vi "acquire_ShootDualTalonSrx.vi"(8 "error in":errorcluster, 11 "QuadTalonSRXDriveRef":T1={"LeftMasterDriveRef"={"DeviceStatus"={"status"=FALSE, "code"=0, "source"=""}, "Type"=enum."PWM", "PWM"={"PWM Channel"=enum."Invalid", "DeadBand"={"Name"="", "maxPositivePwm"=0, "minPositivePwm"=0, "centerPwm"=0, "maxNegativePwm"=0, "minNegativePwm"=0, "angularRange"=0}}, "CAN"={"Device Number"=0, "SetOutput VI Ref"=variant(refnum<vi> refnum), "GetOutput VI Ref"=variant(refnum<vi> refnum), "Enable VI Ref"=variant(refnum<vi> refnum), "Disable VI Ref"=variant(refnum<vi> refnum), "Data"=variant}, "Invert"=FALSE, "DIO PWM"={"PWM \"Enable\" Channel"=enum."Invalid", "DIOChannel"=enum."Invalid", "PWM Rate"=0.0}}, "RightMasterDriveRef"={"DeviceStatus"={"status"=FALSE, "code"=0, "source"=""}, "Type"=enum."PWM", "PWM"={"PWM Channel"=enum."Invalid", "DeadBand"={"Name"="", "maxPositivePwm"=0, "minPositivePwm"=0, "centerPwm"=0, "maxNegativePwm"=0, "minNegativePwm"=0, "angularRange"=0}}, "CAN"={"Device Number"=0, "SetOutput VI Ref"=variant(refnum<vi> refnum), "GetOutput VI Ref"=variant(refnum<vi> refnum), "Enable VI Ref"=variant(refnum<vi> refnum), "Disable VI Ref"=variant(refnum<vi> refnum), "Data"=variant}, "Invert"=FALSE, "DIO PWM"={"PWM \"Enable\" Channel"=enum."Invalid", "DIOChannel"=enum."Invalid", "PWM Rate"=0.0}}}) -> (0 "error out":errorcluster)   [LabVIEW 2019, in "ShootDualTalonSRX_Motor_Pair.lvlib"]
doc: "This VI is called for each TeleOp packet received from the DS where the robot is not disabled. It is often used to read from the joysticks and update I/O or to update setpoints for timed control loops. It should complete and return within 20 milliseconds or it may miss DS packets."
uses:
  ShootDualTalonSRX_Motor_Pair.lvlib
  <vilib>/Rock Robotics/WPI/ThirdParty/Phoenix-LabVIEW/Motor Controller/Get/CTRE_Phoenix_MotorController_GetSelectedSensorData.vi
  <vilib>/Rock Robotics/WPI/ThirdParty/Phoenix-LabVIEW/Motor Controller/Get/CTRE_Phoenix_MotorController_GetVoltage.vi
  globals_ShootDualTalonSRX.vi
  <vilib>/Rock Robotics/SystemInterfaces/DIO/FPGA_DIOPWMChannel.ctl
  <vilib>/Rock Robotics/WPI/PWM/WPI_PWMDeadband.ctl
  <vilib>/Rock Robotics/WPI/MotorControl/WPI_MotorControlType.ctl
  <vilib>/Rock Robotics/SystemInterfaces/DIO/FPGA_DIOChannel.ctl
  <vilib>/Rock Robotics/WPI/MotorControl/WPI_MotorControlDeviceRef.ctl
  ctrlRef_ShootDualTalon.ctl
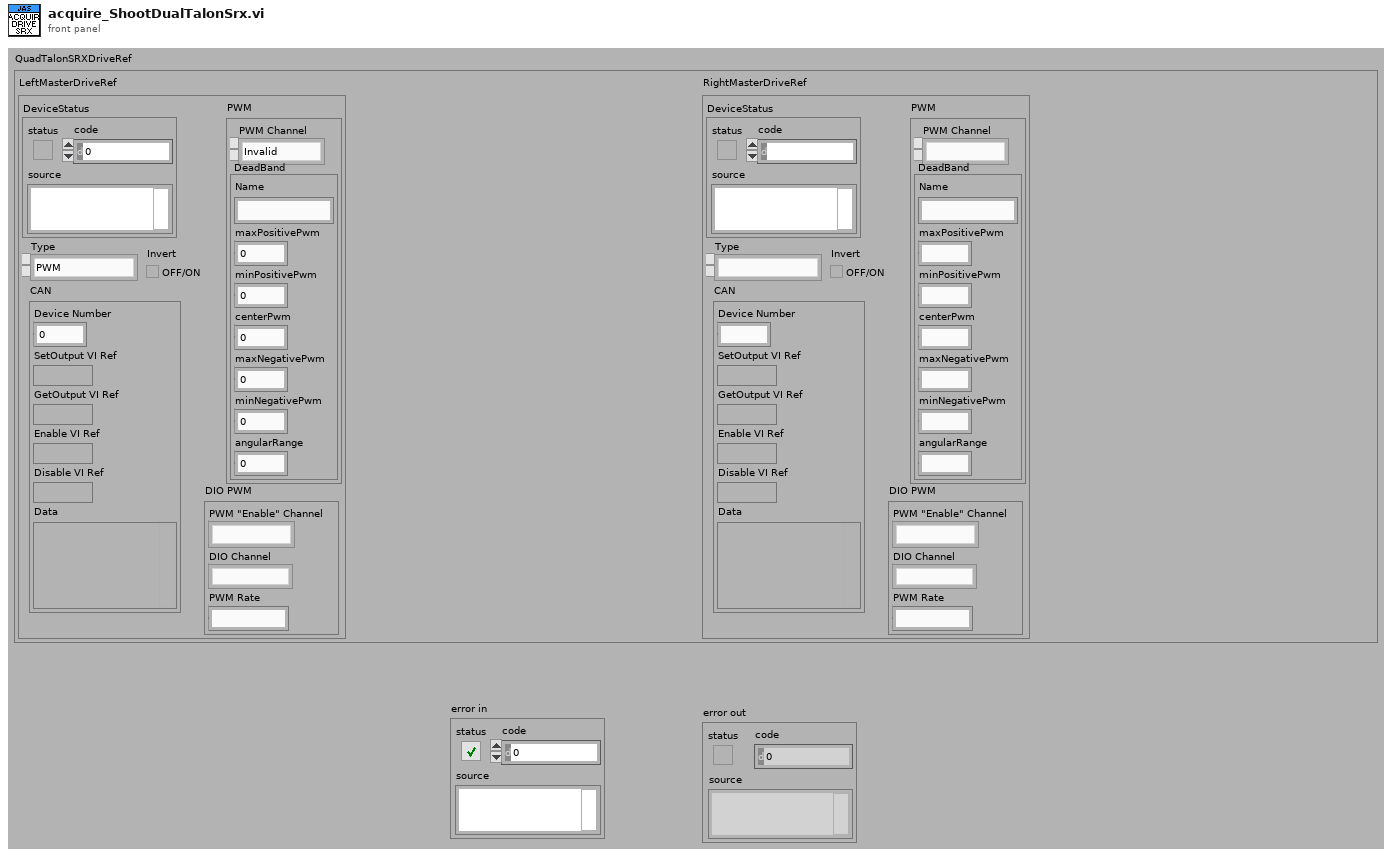
[diagram p1: front panel]
types:
  T1 = typedef "ShootDualTalonSRX_Motor_Pair.lvlib/ctrlRef_ShootDualTalon.ctl" = cluster{"LeftMasterDriveRef":T2, "RightMasterDriveRef":T2}
  T2 = typedef "WPI_MotorControlDeviceRef.ctl" = cluster{"DeviceStatus":errorcluster, "Type":T3, "PWM":cluster{"PWM Channel":T4, "DeadBand":T5}, "CAN":cluster{"Device Number":u8, "SetOutput VI Ref":variant, "GetOutput VI Ref":variant, "Enable VI Ref":variant, "Disable VI Ref":variant, "Data":variant}, "Invert":bool, "DIO PWM":cluster{"PWM \"Enable\" Channel":T4, "DIOChannel":T6, "PWM Rate":dbl}}
  T3 = typedef "WPI_MotorControlType.ctl" = enum16{"PWM", "CAN", "DIO PWM"}
  T4 = typedef "FPGA_DIOPWMChannel.ctl" = enum8{"PWM 0", "PWM 1", "PWM 2", "PWM 3", "PWM 4", "PWM 5", "PWM 6", "PWM 7", "PWM 8", "PWM 9", "PWM MXP 0", "PWM MXP 1", "PWM MXP 2", "PWM MXP 3", "PWM MXP 4", "PWM MXP 5", "PWM MXP 6", "PWM MXP 7", "PWM MXP 8", "PWM MXP 9", "Invalid"}
  T5 = typedef "WPI_PWMDeadband.ctl" = cluster{"Name":string, "maxPositivePwm":i32, "minPositivePwm":i32, "centerPwm":i32, "maxNegativePwm":i32, "minNegativePwm":i32, "angularRange":u16}
  T6 = typedef "FPGA_DIOChannel.ctl" = enum8{"DIO 0", "DIO 1", "DIO 2", "DIO 3", "DIO 4", "DIO 5", "DIO 6", "DIO 7", "DIO 8", "DIO 9", "DIO MXP 0", "DIO MXP 1", "DIO MXP 2", "DIO MXP 3", "DIO MXP 4", "DIO MXP 5", "DIO MXP 6", "DIO MXP 7", "DIO MXP 8", "DIO MXP 9", "DIO MXP 10", "DIO MXP 11", "DIO MXP 12", "DIO MXP 13", "DIO MXP 14", "DIO MXP 15", "SPI Port CS1", "SPI Port CS2", "SPI Port CS3", "SPI Port MISO", "SPI Port MOSI", "Invalid"}
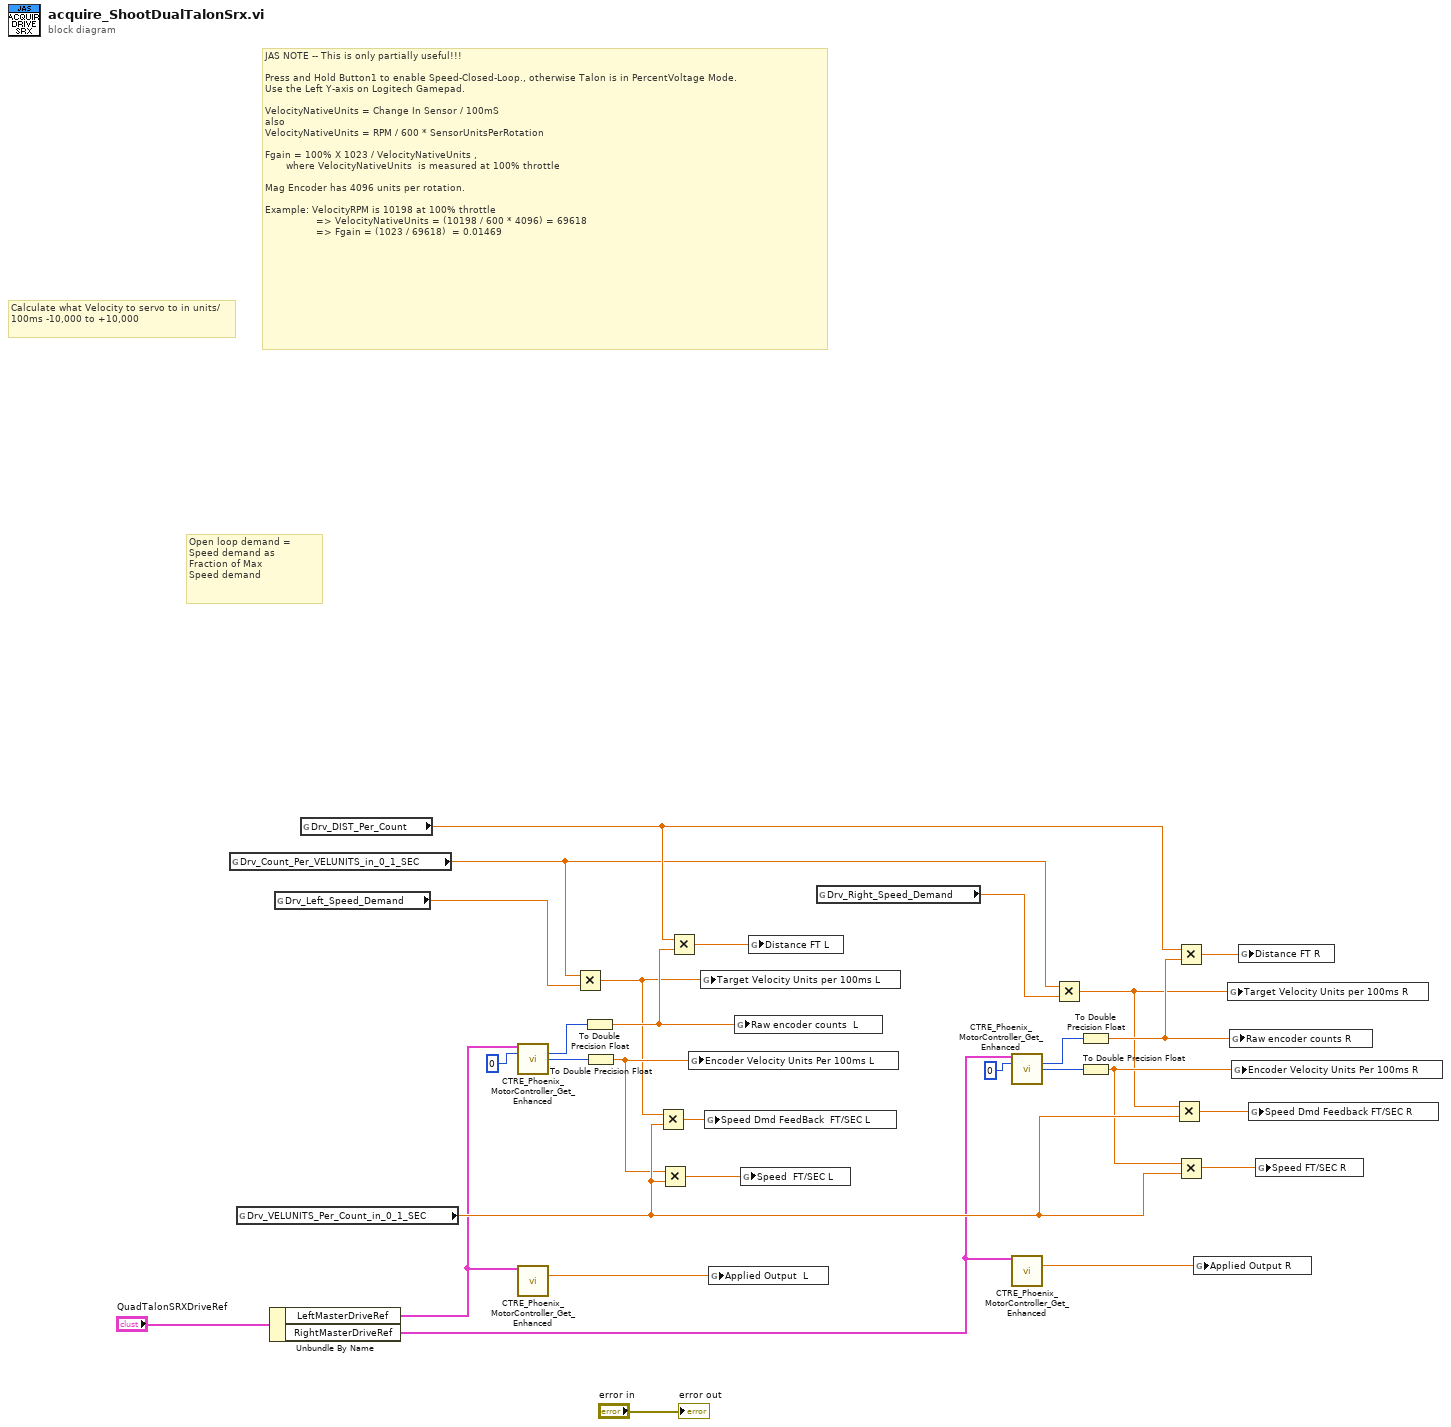
[diagram p0: block diagram]
diagram:
  # "Open loop demand = \nSpeed demand as\nFraction of Max\nSpeed demand"
  # "JAS NOTE -- This is only partially useful!!!\n\nPress and Hold Button1 to enable Speed-Closed-Loop., otherwise Talon is in PercentVoltage Mode.  \nUse the Left Y-axis on Logitech Gamepad.\n\nVelocityNativeUnits = Change In Sensor / 100mS\nalso\nVelocityNativeUnits = RPM / 600 * SensorUnitsPerRotation\n\nFgain = 100% X 1023 / VelocityNativeUnits , \n       where VelocityNativeUnits  is measured at 100% throttle\n\nMag Encoder has 4096 units per rotation.\n\nExample: VelocityRPM is 10198 at 100% throttle\n                 => VelocityNativeUnits = (10198 / 600 * 4096) = 69618\n                 => Fgain = (1023 / 69618)  = 0.01469"
  # "Calculate what Velocity to servo to in units/100ms -10,000 to +10,000"
  n1 = global read "globals_ShootDualTalonSRX.vi" "Drv_Count_Per_VELUNITS_in_0_1_SEC"() -> (w17:dbl)
  n2 = global read "globals_ShootDualTalonSRX.vi" "Drv_VELUNITS_Per_Count_in_0_1_SEC"() -> (w21:dbl)
  n3 = Unbundle By Name("QuadTalonSRXDriveRef") -> ("LeftMasterDriveRef"=w20:T2, "RightMasterDriveRef"=w19:T2)
  n4 = global read "globals_ShootDualTalonSRX.vi" "Drv_Left_Speed_Demand"() -> (w18:dbl)
  n5 = global read "globals_ShootDualTalonSRX.vi" "Drv_DIST_Per_Count"() -> (w22:dbl)
  n6 = call-poly <vilib>:"CTRE_Phoenix_MotorController_Get_Enhanced.vi"("PhoenixMotorControlDevRef"=w20, "pidLoopIdx"=u32 0) -> ("Position (Raw Sensor Units)"=w24:i32, "Velocity (Raw Sensor Units per 100 ms)"=w28:i32)  [unwired: 10 in, 2 out]
  n7 = call-poly <vilib>:"CTRE_Phoenix_MotorController_Get_Enhanced.vi"("PhoenixMotorControlDevRef"=w20) -> ("Percent Output"=w15:dbl)  [unwired: 10 in, 4 out]
  n8 = Multiply(x=w17, y=w18) -> (x*y=w4:dbl)
  n9 = To Double Precision Float(number=w24) -> (double precision float=w6:dbl)
  n10 = To Double Precision Float(number=w28) -> (double precision float=w8:dbl)
  n11 = Multiply(x=w4, y=w21) -> (x*y=w12:dbl)
  n12 = Multiply(x=w8, y=w21) -> (x*y=w13:dbl)
  n13 = Multiply(x=w22, y=w6) -> (x*y=w2:dbl)
  n14 = global write "globals_ShootDualTalonSRX.vi" "Encoder Velocity Units Per 100ms L"(w8) -> ()
  n15 = global write "globals_ShootDualTalonSRX.vi" "Target Velocity Units per 100ms L"(w4) -> ()
  n16 = global write "globals_ShootDualTalonSRX.vi" "Speed Dmd FeedBack  FT/SEC L"(w12) -> ()
  n17 = global write "globals_ShootDualTalonSRX.vi" "Applied Output  L"(w15) -> ()
  n18 = global write "globals_ShootDualTalonSRX.vi" "Raw encoder counts  L"(w6) -> ()
  n19 = global write "globals_ShootDualTalonSRX.vi" "Speed  FT/SEC L"(w13) -> ()
  n20 = global write "globals_ShootDualTalonSRX.vi" "Distance FT L"(w2) -> ()
  n21 = global read "globals_ShootDualTalonSRX.vi" "Drv_Right_Speed_Demand"() -> (w16:dbl)
  n22 = call-poly <vilib>:"CTRE_Phoenix_MotorController_Get_Enhanced.vi"("PhoenixMotorControlDevRef"=w19, "pidLoopIdx"=u32 0) -> ("Position (Raw Sensor Units)"=w23:i32, "Velocity (Raw Sensor Units per 100 ms)"=w26:i32)  [unwired: 10 in, 2 out]
  n23 = call-poly <vilib>:"CTRE_Phoenix_MotorController_Get_Enhanced.vi"("PhoenixMotorControlDevRef"=w19) -> ("Percent Output"=w14:dbl)  [unwired: 10 in, 4 out]
  n24 = Multiply(x=w17, y=w16) -> (x*y=w5:dbl)
  n25 = To Double Precision Float(number=w23) -> (double precision float=w7:dbl)
  n26 = To Double Precision Float(number=w26) -> (double precision float=w9:dbl)
  n27 = Multiply(x=w5, y=w21) -> (x*y=w10:dbl)
  n28 = Multiply(x=w22, y=w7) -> (x*y=w3:dbl)
  n29 = Multiply(x=w9, y=w21) -> (x*y=w11:dbl)
  n30 = global write "globals_ShootDualTalonSRX.vi" "Applied Output R"(w14) -> ()
  n31 = global write "globals_ShootDualTalonSRX.vi" "Target Velocity Units per 100ms R"(w5) -> ()
  n32 = global write "globals_ShootDualTalonSRX.vi" "Raw encoder counts R"(w7) -> ()
  n33 = global write "globals_ShootDualTalonSRX.vi" "Encoder Velocity Units Per 100ms R"(w9) -> ()
  n34 = global write "globals_ShootDualTalonSRX.vi" "Distance FT R"(w3) -> ()
  n35 = global write "globals_ShootDualTalonSRX.vi" "Speed Dmd Feedback FT/SEC R"(w10) -> ()
  n36 = global write "globals_ShootDualTalonSRX.vi" "Speed FT/SEC R"(w11) -> ()
  "error out" <- "error in"
